vi "c ctre phoenixpro request Config Apply.vi"(5 "forceApply":bool, 6 "strlen":u32, 7 "str":string, 8 "error in (no error)":errorcluster, 9 "timeoutSeconds":dbl, 10 "ecuEncoding":u32, 11 "canbus":string) -> (0 "error out":errorcluster, 3 "function return":i32)   [LabVIEW 2020, in "CTRE_PhoenixTools.lvlib"]
doc: "CTREXPORT int c_ctre_phoenixpro_requestConfigApply(const char *canbus, uint32_t ecuEncoding, double timeoutSeconds, const char *str, uint32_t strlen, bool forceApply);"
uses:
  CTRE_PhoenixTools.lvlib
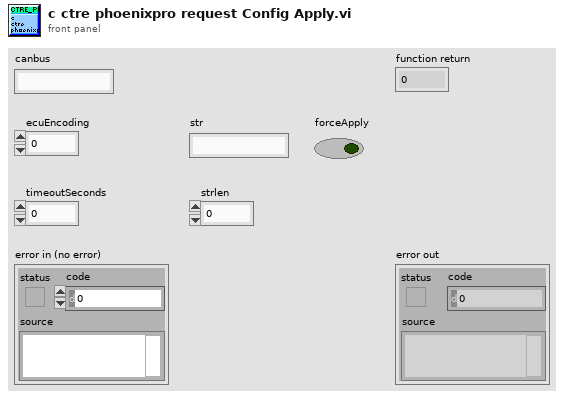
[diagram p1: front panel]
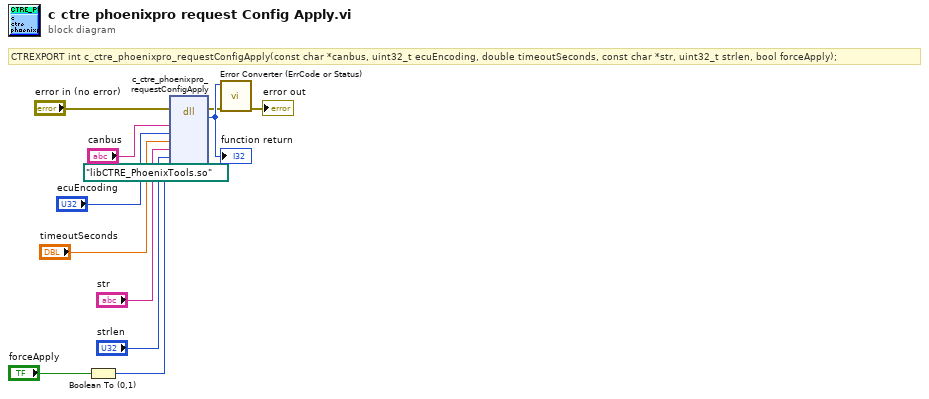
[diagram p0: block diagram]
diagram:
  # "CTREXPORT int c_ctre_phoenixpro_requestConfigApply(const char *canbus, uint32_t ecuEncoding, double timeoutSeconds, const char *str, uint32_t strlen, bool forceApply);"
  n1 = Boolean To (0,1)(Boolean="forceApply") -> (0, 1=w5:i16)
  n2 = dll-call lib="?" fn="c_ctre_phoenixpro_requestConfigApply"(path in=path "libCTRE_PhoenixTools.so", error in="error in (no error)", "canbus"="canbus", "ecuEncoding"="ecuEncoding", "timeoutSeconds"="timeoutSeconds", "str"="str", "strlen"="strlen", "forceApply"=w5) -> (error out=w3:errorcluster, w12:i32)  [unwired: 7 in, 1 out]
  "function return" <- w12
  n3 = call "Error Converter (ErrCode or Status).vi"("error in (no error)"=w3, "error code"=w12) -> ("error out"=→"error out":errorcluster)  [unwired: 9 in]
